vi "Set Range.vi"(6 "Control Ref Queue":T1, 8 "error in (no error)":errorcluster, 10 "Multiplot Representation In":T2, 11 "2D Plot.lvclass in":refnum<class "2D Plot.lvclass">) -> (0 "error out":errorcluster, 2 "Multiplot Representation Out":T2, 3 "2D Plot.lvclass out":refnum<class "2D Plot.lvclass">)   [LabVIEW 2020, in "2D Plot.lvclass"]
uses:
  <vilib>/Math Plots/2D Math Plots/2D Plot/2D Plot/2D Plot.lvclass
  <vilib>/Math Plots/2D Math Plots/2D Plot/2D Plot/Typedef/Multiplot Representation.ctl
  <vilib>/Math Plots/2D Math Plots/2D Plot/2D Plot/Typedef/Plot Representation.ctl
  <vilib>/Math Plots/2D Math Plots/2D Plot/2D Plot/Typedef/Range Cluster.ctl
  <vilib>/Math Plots/2D Math Plots/2D Plot/Action String/2DMathPlot Ctrl Act Queue.ctl
  <vilib>/Math Plots/2D Math Plots/2D Plot/Action String/2DMathPlot Ctrl Act Cluster.ctl
  <vilib>/Math Plots/2D Math Plots/2D Plot/Action String/2DMathPlot State Class.ctl
  <vilib>/Math Plots/2D Math Plots/2D Plot/2D Plot/2D Plot.lvclass/2D Plot.ctl
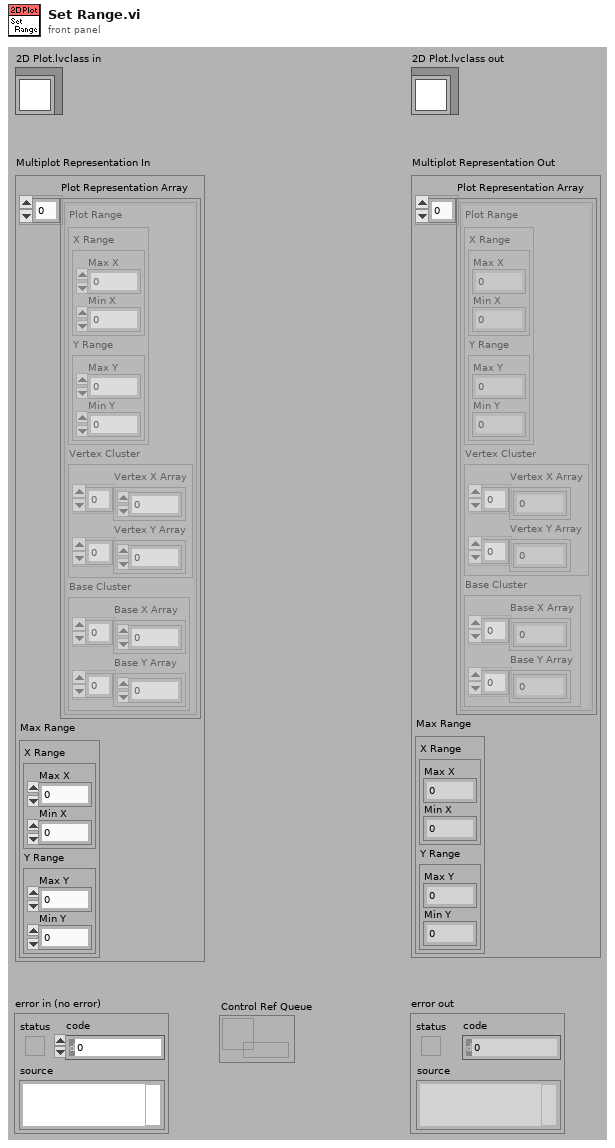
[diagram p1: front panel]
types:
  T1 = typedef "2DMathPlot Ctrl Act Queue.ctl" = refnum<queue>
  T2 = typedef "2D Plot.lvclass/Multiplot Representation.ctl" = cluster{"Plot Representation Array":T3[], "Max Range":T4}
  T3 = typedef "2D Plot.lvclass/Plot Representation.ctl" = cluster{"Plot Range":T4, "Vertex Cluster":cluster{"Vertex X Array":dbl[], "Vertex Y Array":dbl[]}, "Base Cluster":cluster{"Base X Array":dbl[], "Base Y Array":dbl[]}}
  T4 = typedef "2D Plot.lvclass/Range Cluster.ctl" = cluster{"X Range":cluster{"Max X":dbl, "Min X":dbl}, "Y Range":cluster{"Max Y":dbl, "Min Y":dbl}}
  T5 = typedef "2D Plot.lvclass/Scale Array.ctl" = T6[]
  T6 = typedef "2D Plot.lvclass/Scale Cluster.ctl" = cluster{"General":cluster{"Editable":bool, "Flipped":bool, "Mapping Mode":u8, "Visible":bool, "Style":u8, "Scale Fit":u8}, "Offset and Multiplier":T7, "Range":cluster{"Minimum":dbl, "Maximum":dbl, "Increment":dbl, "Minor Increment":dbl, "Start":dbl}, "Tick Color":cluster{"Major Color":u32, "Minor Color":u32}, "Gird Color":cluster{"Major Color":u32, "Minor Color":u32}, "Marker":cluster{"Visible":bool, "FG Color":u32, "BG Color":u32, "Font Name":string, "Font Size":u32, "Font Bold":bool, "Font Italic":bool, "Font Strikeout":bool, "Font Underline":bool}, "Name Label":cluster{"Visible":bool, "FG Color":u32, "BG Color":u32, "Font Name":string, "Font Size":u32, "Font Bold":bool, "Font Italic":bool, "Font Strikeout":bool, "Font Underline":bool, "Justification":enum16{"Left", "Center", "Right"}, "Text":string}}
  T7 = typedef "LVOffsetAndMultiplierTypeDef.ctl" = cluster{"Offset":dbl, "Multiplier":dbl}
  T8 = cluster{"Minimum":dbl, "Maximum":dbl, "Increment":dbl, "Minor Increment":dbl, "Start":dbl}
  T9 = typedef "2DMathPlot Ctrl Act Cluster.ctl" = cluster{"Plot Area Ref":refnum<vi>, "Z Axis Ref":refnum<vi>, "Legend Ref":refnum<vi>, "XControl Ref":refnum<vi>, "Facade Ref":refnum<vi>, "Display State Change Class":T10}
  T10 = typedef "2DMathPlot State Class.ctl" = enum16{"Update All (Undo)", "Update General", "Update Appearance", "Update Format", "Update Scale", "Update Marker", "Update Cursor", "None"}
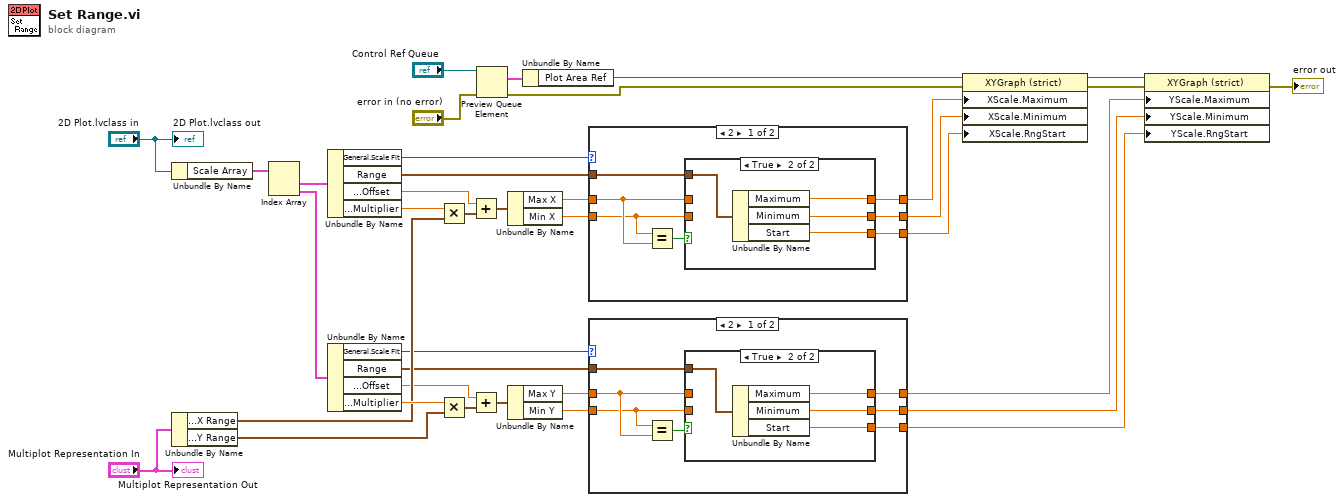
[diagram p0: block diagram]
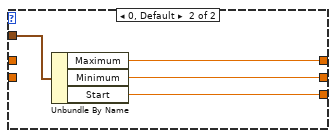
[diagram p3: hidden frame]
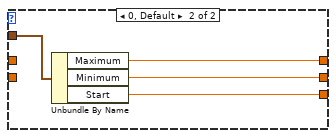
[diagram p5: hidden frame]
diagram:
  n1 = Unbundle By Name("2D Plot.lvclass in") -> ("Scale Array"=w36:T5)
  n2 = Unbundle By Name("Multiplot Representation In") -> ("Max Range.X Range"=w24:cluster{"Max X":dbl, "Min X":dbl}, "Max Range.Y Range"=w26:cluster{"Max Y":dbl, "Min Y":dbl})
  n3 = Index Array(array=w36) -> (element #1=w35:T6, element #2=w34:T6)  [unwired: 2 in]
  n4 = Unbundle By Name(w35) -> ("General.Scale Fit"=w13:u8, "Range"=w33:T8, "Offset and Multiplier.Offset"=w23:dbl, "Offset and Multiplier.Multiplier"=w25:dbl)
  n5 = Unbundle By Name(w34) -> ("General.Scale Fit"=w6:u8, "Range"=w5:T8, "Offset and Multiplier.Offset"=w18:dbl, "Offset and Multiplier.Multiplier"=w27:dbl)
  n6 = Multiply(x=w25, y=w24) -> (x*y=w22:cluster{"Max X":dbl, "Min X":dbl})
  n7 = Multiply(x=w27, y=w26) -> (x*y=w19:cluster{"Max Y":dbl, "Min Y":dbl})
  n8 = Add(x=w23, y=w22) -> (x+y=w21:cluster{"Max X":dbl, "Min X":dbl})
  n9 = Add(x=w18, y=w19) -> (x+y=w17:cluster{"Max Y":dbl, "Min Y":dbl})
  n10 = Preview Queue Element(queue="Control Ref Queue", error in (no error)="error in (no error)") -> (element=w31:T9, error out=w15:errorcluster)  [unwired: 3 out]
  n11 = Unbundle By Name(w21) -> ("Max X"=w14:dbl, "Min X"=w20:dbl)
  n12 = Unbundle By Name(w17) -> ("Max Y"=w4:dbl, "Min Y"=w3:dbl)
  n13 = Unbundle By Name(w31) -> ("Plot Area Ref"=w16:refnum<vi>)
  n14 = case shown="2" w13 {
    tunnel: w33 -> [w43 w54]
    tunnel: w14 -> [w41 _]
    tunnel: w20 -> [w39 _]
    tunnel: [w42 w51] -> w11
    tunnel: [w40 w52] -> w12
    tunnel: [w38 w53] -> w10
    frame 2 {
      n15 = Equal?(x=w39, y=w41) -> (x = y?=w44:bool)
      n16 = case shown="True" w44 {
        tunnel: w43 -> [_ w50]
        tunnel: [w46 w49] -> w42
        tunnel: w41 -> [w46 _]
        tunnel: [w45 w48] -> w40
        tunnel: w39 -> [w45 _]
        tunnel: [w45 w47] -> w38
        frame False {
        }
        frame True {
          n17 = Unbundle By Name(w50) -> ("Maximum"=w49:dbl, "Minimum"=w48:dbl, "Start"=w47:dbl)
        }
      }
    }
    frame 0, Default {
      n18 = Unbundle By Name(w54) -> ("Maximum"=w51:dbl, "Minimum"=w52:dbl, "Start"=w53:dbl)
    }
  }
  n19 = case shown="2" w6 {
    tunnel: w5 -> [w60 w71]
    tunnel: w4 -> [w58 _]
    tunnel: w3 -> [w57 _]
    tunnel: [w59 w68] -> w8
    tunnel: [w56 w69] -> w7
    tunnel: [w55 w70] -> w9
    frame 2 {
      n20 = Equal?(x=w57, y=w58) -> (x = y?=w61:bool)
      n21 = case shown="True" w61 {
        tunnel: w60 -> [_ w67]
        tunnel: [w63 w66] -> w59
        tunnel: w58 -> [w63 _]
        tunnel: w57 -> [w62 _]
        tunnel: [w62 w65] -> w56
        tunnel: [w62 w64] -> w55
        frame False {
        }
        frame True {
          n22 = Unbundle By Name(w67) -> ("Maximum"=w66:dbl, "Minimum"=w65:dbl, "Start"=w64:dbl)
        }
      }
    }
    frame 0, Default {
      n23 = Unbundle By Name(w71) -> ("Maximum"=w68:dbl, "Minimum"=w69:dbl, "Start"=w70:dbl)
    }
  }
  n24 = property class="XYGraph (strict)"(reference=w16, error in=w15, "XScale.Maximum"=w11, "XScale.Minimum"=w12, "XScale.RngStart"=w10) -> (reference out=w2:refnum<vi>, error out=w1:errorcluster)
  n25 = property class="XYGraph (strict)"(reference=w2, error in=w1, "YScale.Maximum"=w8, "YScale.Minimum"=w7, "YScale.RngStart"=w9) -> (error out=→"error out":errorcluster)  [unwired: 1 out]
  "2D Plot.lvclass out" <- "2D Plot.lvclass in"
  "Multiplot Representation Out" <- "Multiplot Representation In"
